vi "digitally_ros_without_joystick_2.vi"() -> ()   [LabVIEW 2019]
uses:
  <vilib>/addons/eal4LabVIEW/ApiLib/Connection control/ealApiConnect_string.vi
  <vilib>/addons/eal4LabVIEW/eal4LabVIEW.lvlib
panel:
  out "Diviation 3":dbl
  out "Diviation 2":dbl
  out "Diviation 1":dbl
  out "Sensor values":dbl[](array[numeric])
  out "List length":i32
  in  "stop 3":bool
  in  "stop 2":bool
  out "I value":i32
  out "error out":errorcluster
  out "Is the PID fnished?":bool[](array[boolean])
  out "In Range? (1)":bool
  out "In Range? (2)":bool
  out "In Range? (3)":bool
  in  "condition 6":i32(ring) items=["AXIS_CONDITION_ACTIVE"=0, "AXIS_CONDITION_PARKING"=1, "AXIS_CONDITION_DEACTIVATED"=2, "AXIS_CONDITION_ACTIVE_DECOUPLED"=4, "AXIS_CONDITION_PARKING_DECOUPLED"=5, "AXIS_CONDITION_DEACTIVATED_DECOUPLED"=6, "AXIS_CONDITION_ACTIVE_PARAMETERIZATION"=8, "AXIS_CONDITION_PARKING_PARAMETERIZATION"=9, "AXIS_CONDITION_DEACTIVATED_PARAMETERIZATION"=10, "AXIS_CONDITION_ACTIVE_DECOUPLED_PARAMETERIZATION"=12, "AXIS_CONDITION_PARKING_DECOUPLED_PARAMETERIZATION"=13, "AXIS_CONDITION_DEACTIVATED_DECOUPLED_PARAMETERIZATION"=14]
  in  "slave index 6":i32
  in  "condition 5":i32(ring) items=["AXIS_CONDITION_ACTIVE"=0, "AXIS_CONDITION_PARKING"=1, "AXIS_CONDITION_DEACTIVATED"=2, "AXIS_CONDITION_ACTIVE_DECOUPLED"=4, "AXIS_CONDITION_PARKING_DECOUPLED"=5, "AXIS_CONDITION_DEACTIVATED_DECOUPLED"=6, "AXIS_CONDITION_ACTIVE_PARAMETERIZATION"=8, "AXIS_CONDITION_PARKING_PARAMETERIZATION"=9, "AXIS_CONDITION_DEACTIVATED_PARAMETERIZATION"=10, "AXIS_CONDITION_ACTIVE_DECOUPLED_PARAMETERIZATION"=12, "AXIS_CONDITION_PARKING_DECOUPLED_PARAMETERIZATION"=13, "AXIS_CONDITION_DEACTIVATED_DECOUPLED_PARAMETERIZATION"=14]
  in  "slave index 5":i32
  in  "condition 4":i32(ring) items=["AXIS_CONDITION_ACTIVE"=0, "AXIS_CONDITION_PARKING"=1, "AXIS_CONDITION_DEACTIVATED"=2, "AXIS_CONDITION_ACTIVE_DECOUPLED"=4, "AXIS_CONDITION_PARKING_DECOUPLED"=5, "AXIS_CONDITION_DEACTIVATED_DECOUPLED"=6, "AXIS_CONDITION_ACTIVE_PARAMETERIZATION"=8, "AXIS_CONDITION_PARKING_PARAMETERIZATION"=9, "AXIS_CONDITION_DEACTIVATED_PARAMETERIZATION"=10, "AXIS_CONDITION_ACTIVE_DECOUPLED_PARAMETERIZATION"=12, "AXIS_CONDITION_PARKING_DECOUPLED_PARAMETERIZATION"=13, "AXIS_CONDITION_DEACTIVATED_DECOUPLED_PARAMETERIZATION"=14]
  in  "slave index 4":i32
  out "RPM 1 ROS":dbl
  out "RPM 2 ROS":dbl
  out "RPM 3 ROS":dbl
  in  "stop 1":bool
  out "Return value":dbl[](array[numeric])
  out "Iteration counter":i32
  # "ROS Control"
  # "Joystick Control"
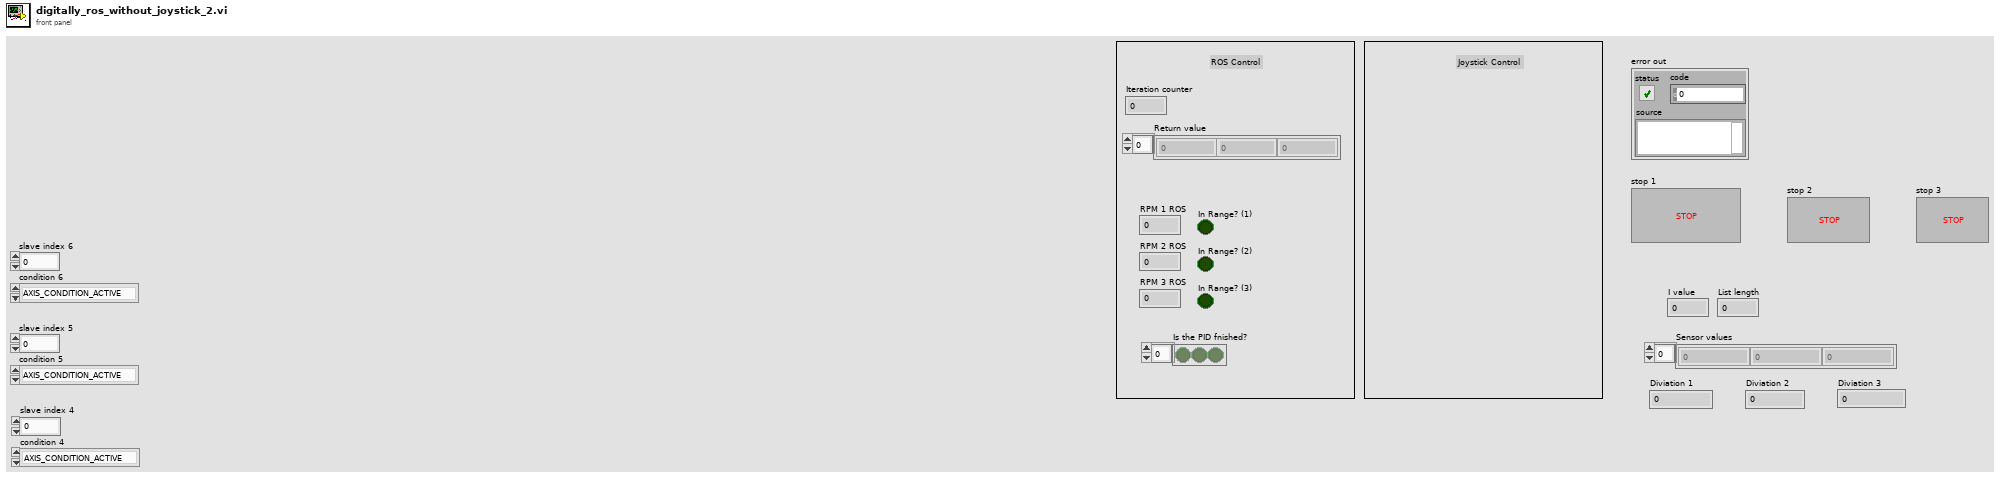
[diagram p1: front panel]
types:
  T1 = cluster{"Velocity":dbl, "Acceleration":dbl, "Deceleration":dbl, "Jerk":dbl}
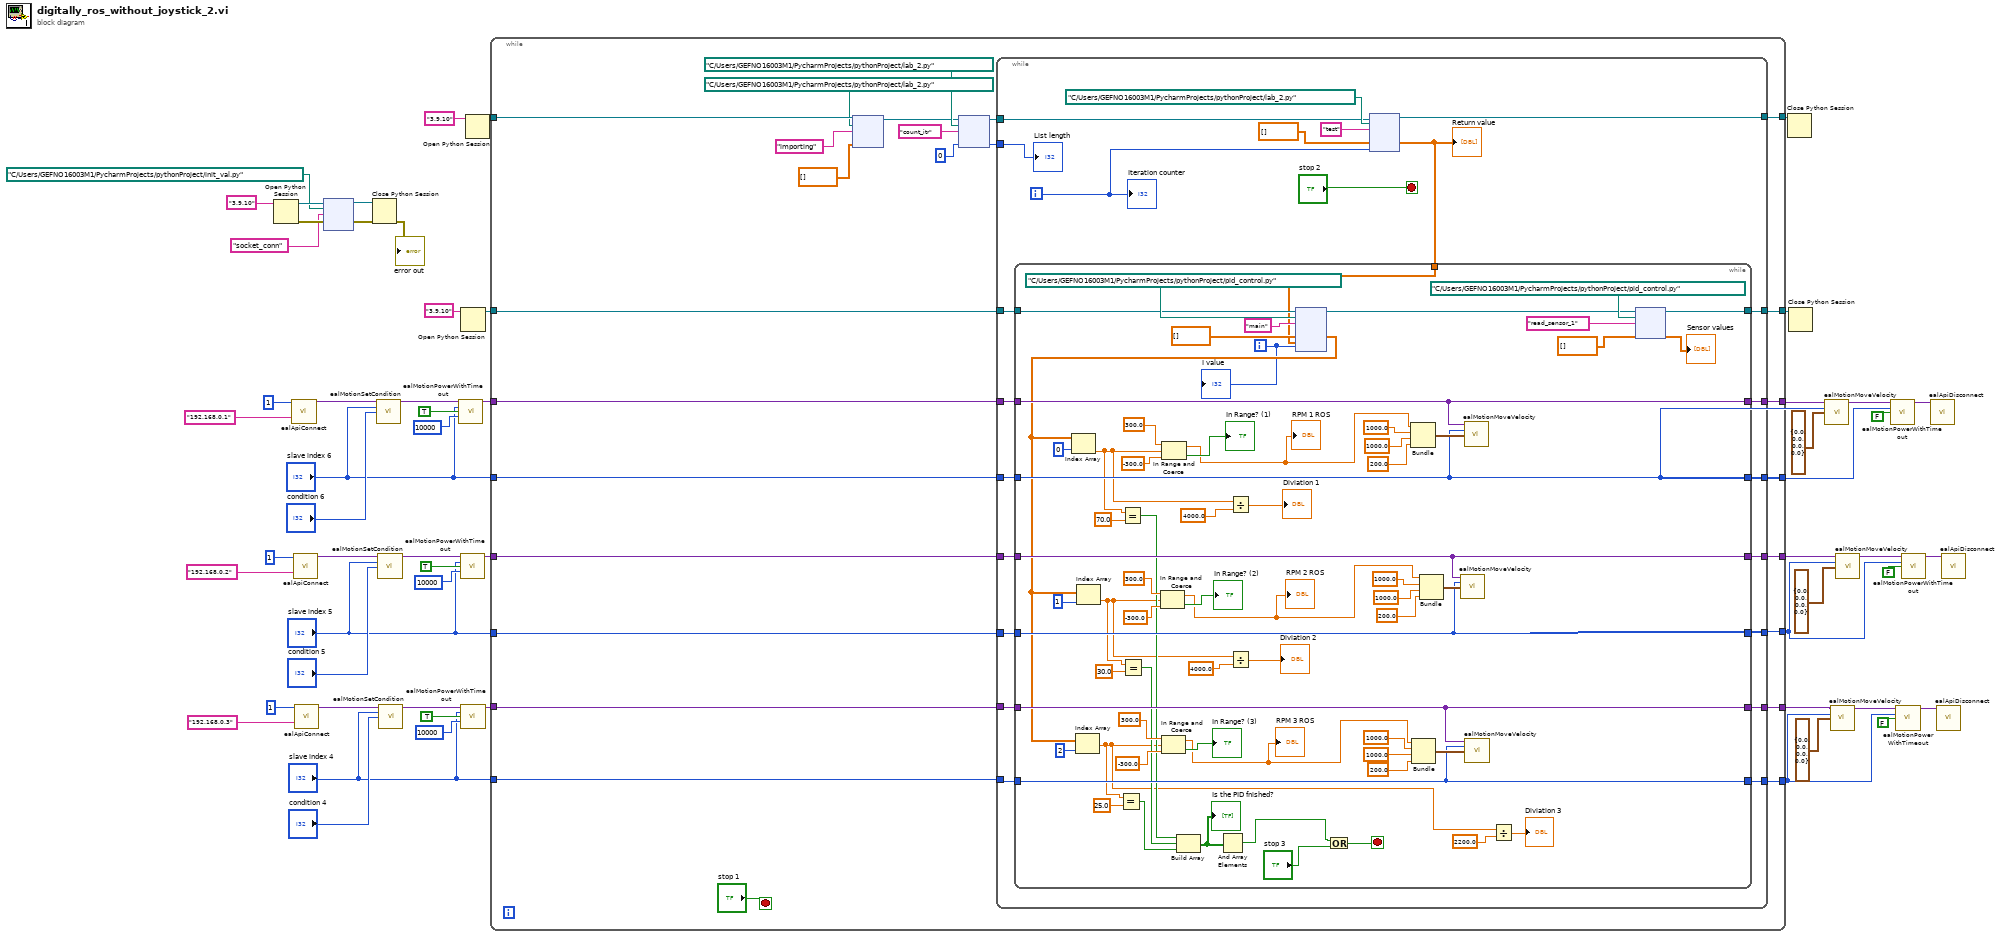
[diagram p0: block diagram]
diagram:
  n1 = Open Python Session(python version="3.9.10" ("Python version")) -> (session out=w8:refnum<k35>, error out=w6:errorcluster)  [unwired: 2 in]
  n2 = call-poly <vilib>:"ealApiConnect.vi"("maximum no of axes"=1, "ip address"="192.168.0.1") -> ("connection out"=w31:variant)  [unwired: 12 in, 1 out]
  n3 = call-poly <vilib>:"ealApiConnect.vi"("maximum no of axes"=1, "ip address"="192.168.0.2") -> ("connection out"=w38:variant)  [unwired: 12 in, 1 out]
  n4 = call-poly <vilib>:"ealApiConnect.vi"("maximum no of axes"=1, "ip address"="192.168.0.3") -> ("connection out"=w45:variant)  [unwired: 12 in, 1 out]
  n5 = node(w8, path "C:/Users/GEFNO16003M1/PycharmProjects/pythonProject/init_val.py" ("module path"), "socket_conn" ("function name"), w6) -> (w7:refnum<k35>, w5:errorcluster)  [unwired: 2 in, 2 out]
  n6 = Close Python Session(session in=w7, error in=w5) -> (11:→"error out":errorcluster)
  n7 = call <vilib>:"ealMotionSetCondition.vi"("connection in"=w31, "slave index"="slave index 6", "condition"="condition 6") -> ("connection out"=w30:variant)  [unwired: 11 in, 1 out]
  n8 = call <vilib>:"ealMotionSetCondition.vi"("connection in"=w38, "slave index"="slave index 5", "condition"="condition 5") -> ("connection out"=w37:variant)  [unwired: 11 in, 1 out]
  n9 = call <vilib>:"ealMotionSetCondition.vi"("connection in"=w45, "slave index"="slave index 4", "condition"="condition 4") -> ("connection out"=w44:variant)  [unwired: 11 in, 1 out]
  n10 = call <vilib>:"ealMotionPowerWithTimeout.vi"("connection in"=w30, "slave index"="slave index 6", "value"=TRUE, "timeout"=10000) -> ("connection out"=w26:variant)  [unwired: 10 in, 1 out]
  n11 = call <vilib>:"ealMotionPowerWithTimeout.vi"("connection in"=w37, "slave index"="slave index 5", "value"=TRUE, "timeout"=10000) -> ("connection out"=w25:variant)  [unwired: 10 in, 1 out]
  n12 = Open Python Session(python version="3.9.10" ("Python version")) -> (session out=w12:refnum<k35>)  [unwired: 2 in, 1 out]
  n13 = call <vilib>:"ealMotionPowerWithTimeout.vi"("connection in"=w44, "slave index"="slave index 4", "value"=TRUE, "timeout"=10000) -> ("connection out"=w24:variant)  [unwired: 10 in, 1 out]
  n14 = Open Python Session(python version="3.9.10" ("Python version")) -> (session out=w15:refnum<k35>)  [unwired: 2 in, 1 out]
  n15 = while {
    tunnel: w26 -> [w84]
    tunnel: w25 -> [w83]
    tunnel: w24 -> [w82]
    tunnel: [w69] -> w23
    tunnel: [w81] -> w22
    tunnel: "slave index 6" -> [w80]
    tunnel: "slave index 5" -> [w79]
    tunnel: [w78] -> w19
    tunnel: [w72] -> w18
    tunnel: "slave index 4" -> [w77]
    tunnel: w15 -> [w76]
    tunnel: [w75] -> w14
    tunnel: w12 -> [w74]
    tunnel: [w70] -> w11
    tunnel: [w73] -> w10
    tunnel: [w71] -> w9
    stop <- "stop 1" stop-if-true
    n16 = node(w76, path "C:/Users/GEFNO16003M1/PycharmProjects/pythonProject/lab_2.py" ("module path"), "importing" ("function name"), dbl[] []) -> (w63:refnum<k35>)  [unwired: 2 in, 3 out]
    n17 = node(w63, path "C:/Users/GEFNO16003M1/PycharmProjects/pythonProject/lab_2.py" ("module path"), "count_itr" ("function name"), 0) -> (w62:refnum<k35>, w60:i32)  [unwired: 1 in, 3 out]
    n18 = while {
      tunnel: [w104] -> w75
      tunnel: w62 -> [w106]
      tunnel: w60 -> [w86]
      tunnel: w84 -> [w102]
      tunnel: w83 -> [w91]
      tunnel: w82 -> [w101]
      tunnel: [w93] -> w69
      tunnel: [w94] -> w81
      tunnel: w80 -> [w92]
      tunnel: w79 -> [w90]
      tunnel: [w95] -> w78
      tunnel: w77 -> [w97]
      tunnel: w74 -> [w89]
      tunnel: [w99] -> w70
      tunnel: [w98] -> w73
      tunnel: [w96] -> w72
      tunnel: [w88] -> w71
      i -> [w100]
      stop <- "stop 2" stop-if-true
      n19 = node(w106, path "C:/Users/GEFNO16003M1/PycharmProjects/pythonProject/lab_2.py" ("module path"), "test" ("function name"), dbl[] [], w100) -> (w104:refnum<k35>, w103:dbl[])  [unwired: 2 in, 3 out]
      "Return value" <- w103
      n20 = while {
        tunnel: w103 -> [w124]
        tunnel: w102 -> [w144]
        tunnel: w101 -> [w146]
        tunnel: [w146] -> w99
        tunnel: [w145] -> w98
        tunnel: w97 -> [w145]
        tunnel: [w142] -> w96
        tunnel: [w141] -> w95
        tunnel: [w143] -> w94
        tunnel: [w144] -> w93
        tunnel: w92 -> [w143]
        tunnel: w91 -> [w142]
        tunnel: w90 -> [w141]
        tunnel: w89 -> [w140]
        tunnel: [w123] -> w88
        i -> [w128]
        stop <- w127 stop-if-true
        n21 = node(w140, path "C:/Users/GEFNO16003M1/PycharmProjects/pythonProject/pid_control.py" ("module path"), "main" ("function name"), dbl[] [], w124, w128) -> (w118:refnum<k35>, w139:dbl[])  [unwired: 3 in, 3 out]
        n22 = Index Array(array=w139, index=0) -> (element=w117:dbl)
        n23 = Index Array(array=w139, index=2) -> (element=w111:dbl)
        n24 = Index Array(array=w139, index=1) -> (element=w114:dbl)
        n25 = Equal?(x=w111, y=25.0) -> (x = y?=w133:bool)
        n26 = Equal?(x=w117, y=70.0) -> (x = y?=w135:bool)
        n27 = Equal?(x=w114, y=30.0) -> (x = y?=w134:bool)
        n28 = In Range and Coerce(upper limit=300.0, x=w114, lower limit=-300.0) -> (coerced(x)=w130:dbl, In Range?=→"In Range? (2)":bool)
        "RPM 2 ROS" <- w130
        n29 = In Range and Coerce(upper limit=300.0, x=w111, lower limit=-300.0) -> (coerced(x)=w129:dbl, In Range?=→"In Range? (3)":bool)
        "RPM 3 ROS" <- w129
        n30 = In Range and Coerce(upper limit=300.0, x=w117, lower limit=-300.0) -> (coerced(x)=w131:dbl, In Range?=→"In Range? (1)":bool)
        "RPM 1 ROS" <- w131
        n31 = Build Array(w135, w134, w133) -> (w132:bool[])
        "Is the PID fnished?" <- w132
        n32 = And Array Elements(Boolean array=w132) -> (logical AND=w126:bool)
        n33 = Divide(x=w117, y=4000.0) -> (x/y=→"Diviation 1":dbl)
        n34 = Divide(x=w114, y=4000.0) -> (x/y=→"Diviation 2":dbl)
        n35 = Or(x=w126, y="stop 3") -> (x .or. y?=w127:bool)
        n36 = Bundle("upper limit"=w131, 1000.0, 1000.0, 200.0) -> (w156:cluster{"upper limit":dbl, dbl, dbl, dbl})  [unwired: 1 in]
        n37 = Bundle("upper limit"=w129, 1000.0, 1000.0, 200.0) -> (w166:cluster{"upper limit":dbl, dbl, dbl, dbl})  [unwired: 1 in]
        n38 = Bundle("upper limit"=w130, 1000.0, 1000.0, 200.0) -> (w161:cluster{"upper limit":dbl, dbl, dbl, dbl})  [unwired: 1 in]
        n39 = call <vilib>:"ealMotionMoveVelocity.vi"("connection in"=w142, "slave index"=w141, "parameters set"=w161) -> ()  [unwired: 11 in, 2 out]
        n40 = call <vilib>:"ealMotionMoveVelocity.vi"("connection in"=w144, "slave index"=w143, "parameters set"=w156) -> ()  [unwired: 11 in, 2 out]
        n41 = call <vilib>:"ealMotionMoveVelocity.vi"("connection in"=w146, "slave index"=w145, "parameters set"=w166) -> ()  [unwired: 11 in, 2 out]
        n42 = Divide(x=w111, y=2200.0) -> (x/y=→"Diviation 3":dbl)
        n43 = node(w118, path "C:/Users/GEFNO16003M1/PycharmProjects/pythonProject/pid_control.py" ("module path"), "read_sensor_1" ("function name"), dbl[] []) -> (w123:refnum<k35>, →"Sensor values":dbl[])  [unwired: 1 in, 3 out]
        "I value" <- w128
      }
      "Iteration counter" <- w100
      "List length" <- w86
    }
  }
  n44 = Close Python Session(session in=w14) -> ()  [unwired: 1 in, 1 out]
  n45 = Close Python Session(session in=w9) -> ()  [unwired: 1 in, 1 out]
  n46 = call <vilib>:"ealMotionMoveVelocity.vi"("connection in"=w23, "slave index"=w22, "parameters set"=T1 {"Velocity"=0.0, "Acceleration"=0.0, "Deceleration"=0.0, "Jerk"=0.0}) -> ("connection out"=w50:variant)  [unwired: 11 in, 1 out]
  n47 = call <vilib>:"ealMotionMoveVelocity.vi"("connection in"=w11, "slave index"=w10, "parameters set"=T1 {"Velocity"=0.0, "Acceleration"=0.0, "Deceleration"=0.0, "Jerk"=0.0}) -> ("connection out"=w58:variant)  [unwired: 11 in, 1 out]
  n48 = call <vilib>:"ealMotionMoveVelocity.vi"("connection in"=w18, "slave index"=w19, "parameters set"=T1 {"Velocity"=0.0, "Acceleration"=0.0, "Deceleration"=0.0, "Jerk"=0.0}) -> ("connection out"=w54:variant)  [unwired: 11 in, 1 out]
  n49 = call <vilib>:"ealMotionPowerWithTimeout.vi"("connection in"=w50, "slave index"=w22, "value"=FALSE) -> ("connection out"=w51:variant)  [unwired: 11 in, 1 out]
  n50 = call <vilib>:"ealMotionPowerWithTimeout.vi"("connection in"=w58, "slave index"=w10, "value"=FALSE) -> ("connection out"=w59:variant)  [unwired: 11 in, 1 out]
  n51 = call <vilib>:"ealMotionPowerWithTimeout.vi"("connection in"=w54, "slave index"=w19, "value"=FALSE) -> ("connection out"=w55:variant)  [unwired: 11 in, 1 out]
  n52 = call <vilib>:"ealApiDisconnect.vi"("connection in"=w51) -> ()  [unwired: 14 in, 1 out]
  n53 = call <vilib>:"ealApiDisconnect.vi"("connection in"=w59) -> ()  [unwired: 14 in, 1 out]
  n54 = call <vilib>:"ealApiDisconnect.vi"("connection in"=w55) -> ()  [unwired: 14 in, 1 out]
